vi "RPM to Radians per Second (Scalar).vi"(3 "rpm":dbl) -> (1 "radians per second":dbl)   [LabVIEW 2017, in "NI_Robotics Utilities.lvlib"]
doc: "Converts an angular velocity from rpm to radians per second."
uses:
  <vilib>/robotics/Utilities/NI_Robotics Utilities.lvlib
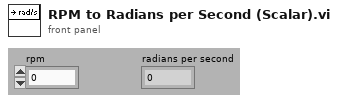
[diagram p1: front panel]
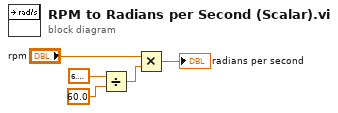
[diagram p0: block diagram]
diagram:
  n1 = Divide(x=6.283185307179586, y=60.0 ("x")) -> (x/y=w4:dbl)
  n2 = Multiply(x="rpm", y=w4) -> (x*y=→"radians per second":dbl)
